vi "io.vi"() -> ()   [LabVIEW 2019]
panel:
  in  "Button 2":bool
  in  "Tab Control":enum32{"IO", "PWM", "I2C"}(tab)
  in  "D14":bool
  in  "D13":bool
  in  "D12":bool
  in  "D11":bool
  in  "D10":bool
  in  "D9":bool
  in  "D8":bool
  in  "D7":bool
  in  "D6":bool
  in  "D5":bool
  in  "D4":bool
  in  "D3":bool
  in  "D2":bool
  in  "D1":bool
  in  "D1 2":bool
  in  "D2 2":bool
  in  "D3 2":bool
  in  "D4 2":bool
  in  "D5 2":bool
  in  "D6 2":bool
  in  "D7 2":bool
  in  "D8 2":bool
  in  "D9 2":bool
  in  "D10 2":bool
  in  "D11 2":bool
  in  "D12 2":bool
  in  "D13 2":bool
  in  "D14 2":bool
  in  "Button":bool
  in  "element":dbl
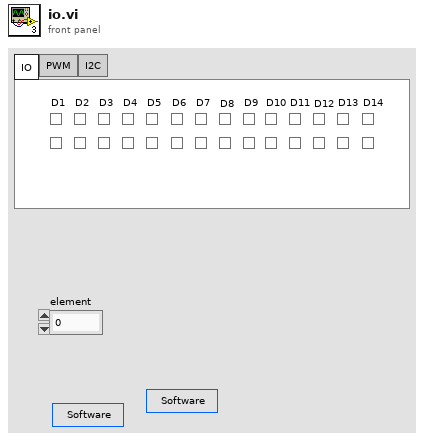
[diagram p1: front panel]
types:
  T1 = enum8{"Enabled", "Disabled", "Disabled and Grayed Out"}
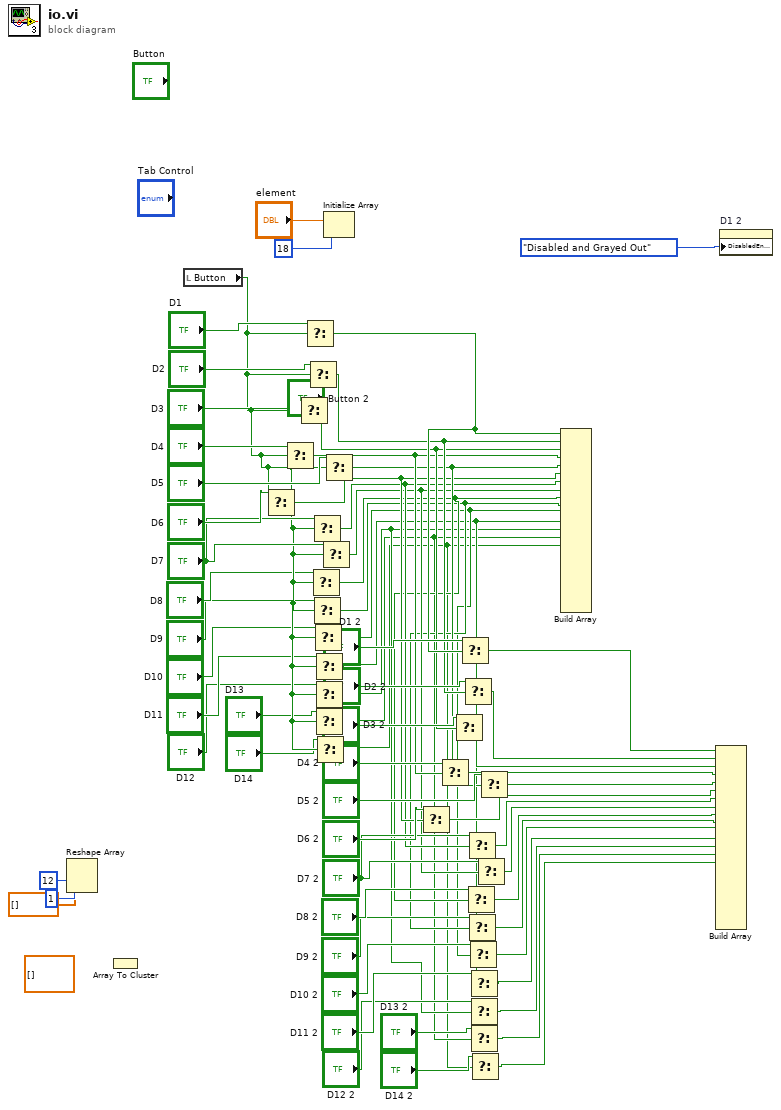
[diagram p0: block diagram]
diagram:
  (unwired) dbl[][] [] ("output array")
  n1 = Reshape Array(dbl[] [] ("array"), 12 ("dimension size"), 1 ("dimension size")) -> ()  [unwired: 1 out]
  n2 = Array To Cluster() -> ()  [unwired: 1 in, 1 out]
  n3 = local read "Button"() -> (w56:bool)
  n4 = Select(t="D6", s=w56) -> (s? t:f=w15:bool)  [unwired: 1 in]
  n5 = Select(t="D4", s=w56) -> (s? t:f=w17:bool)  [unwired: 1 in]
  n6 = Select(t="D3", s=w56) -> (s? t:f=w18:bool)  [unwired: 1 in]
  n7 = Select(t="D1", s=w56) -> (s? t:f=w20:bool)  [unwired: 1 in]
  n8 = Select(t="D2", s=w56) -> (s? t:f=w19:bool)  [unwired: 1 in]
  n9 = Select(t="D8", s=w56) -> (s? t:f=w12:bool)  [unwired: 1 in]
  n10 = Select(t="D7", s=w56) -> (s? t:f=w14:bool)  [unwired: 1 in]
  n11 = Select(t="D9", s=w56) -> (s? t:f=w11:bool)  [unwired: 1 in]
  n12 = Select(t="D10", s=w56) -> (s? t:f=w10:bool)  [unwired: 1 in]
  n13 = Select(t="D11", s=w56) -> (s? t:f=w9:bool)  [unwired: 1 in]
  n14 = Select(t="D12", s=w56) -> (s? t:f=w8:bool)  [unwired: 1 in]
  n15 = Select(t="D13", s=w56) -> (s? t:f=w7:bool)  [unwired: 1 in]
  n16 = Select(t="D14", s=w56) -> (s? t:f=w6:bool)  [unwired: 1 in]
  n17 = Select(t="D7", s=w56) -> (s? t:f=w13:bool)  [unwired: 1 in]
  n18 = Initialize Array("element", 18 ("dimension size")) -> ()  [unwired: 1 out]
  n19 = Select(t="D5", s=w56) -> (s? t:f=w16:bool)  [unwired: 1 in]
  n20 = Select(t="D6 2", s=w15) -> (s? t:f=w38:bool)  [unwired: 1 in]
  n21 = Select(t="D4 2", s=w17) -> (s? t:f=w44:bool)  [unwired: 1 in]
  n22 = Select(t="D3 2", s=w18) -> (s? t:f=w45:bool)  [unwired: 1 in]
  n23 = Select(t="D1 2", s=w20) -> (s? t:f=w1:bool)  [unwired: 1 in]
  n24 = Select(t="D2 2", s=w19) -> (s? t:f=w47:bool)  [unwired: 1 in]
  n25 = Select(t="D8 2", s=w12) -> (s? t:f=w34:bool)  [unwired: 1 in]
  n26 = Select(t="D7 2", s=w14) -> (s? t:f=w37:bool)  [unwired: 1 in]
  n27 = Select(t="D9 2", s=w11) -> (s? t:f=w33:bool)  [unwired: 1 in]
  n28 = Select(t="D10 2", s=w10) -> (s? t:f=w32:bool)  [unwired: 1 in]
  n29 = Select(t="D11 2", s=w9) -> (s? t:f=w31:bool)  [unwired: 1 in]
  n30 = Select(t="D12 2", s=w8) -> (s? t:f=w30:bool)  [unwired: 1 in]
  n31 = Select(t="D13 2", s=w7) -> (s? t:f=w29:bool)  [unwired: 1 in]
  n32 = Select(t="D14 2", s=w6) -> (s? t:f=w28:bool)  [unwired: 1 in]
  n33 = Select(t="D7 2", s=w13) -> (s? t:f=w36:bool)  [unwired: 1 in]
  n34 = Select(t="D5 2", s=w16) -> (s? t:f=w41:bool)  [unwired: 1 in]
  n35 = Build Array(w20, w19, w18, w17, w16, w15, w14, w13, w12, w11, w10, w9, w8, w7, w6) -> ()  [unwired: 8 in, 1 out]
  n36 = Build Array(w1, w47, w45, w44, w41, w38, w37, w36, w34, w33, w32, w31, w30, w29, w28) -> ()  [unwired: 8 in, 1 out]
  n37 = property on="D1 2" class="Bool (strict)"("DisabledEnum"=T1."Disabled and Grayed Out" ("Disabled")) -> ()  [unwired: 2 in, 2 out]
